vi "createNewArrayObject.vi"(8 "error in (no error)":errorcluster, 10 "arrayRef":refnum<vi>, 11 "Enum in":refnum<class "Enum.lvclass">) -> (0 "error out":errorcluster, 3 "Enum out":refnum<class "Enum.lvclass">)   [LabVIEW 2016, in "Enum.lvclass"]
uses:
  Enum.lvclass
  <vilib>/Utility/miscctls.llb/LVPointTypeDef.ctl
  Enum.lvclass/Enum.ctl
panel:
  in  "Enum":enum32{""}(ring)
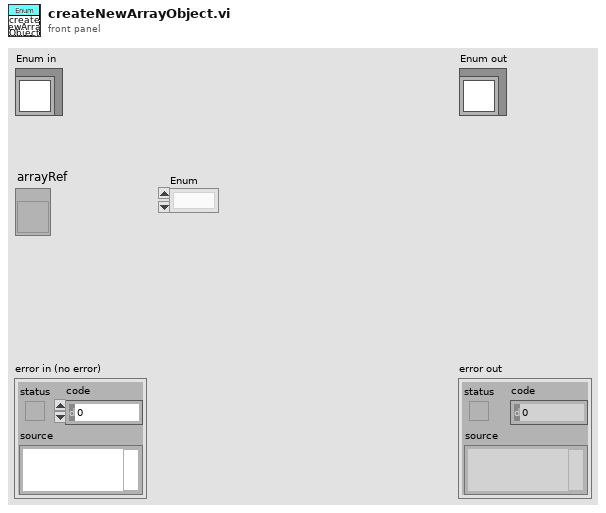
[diagram p1: front panel]
types:
  T1 = typedef "LVPointTypeDef.ctl" = cluster{"Horizontal":i16, "Vertical":i16}
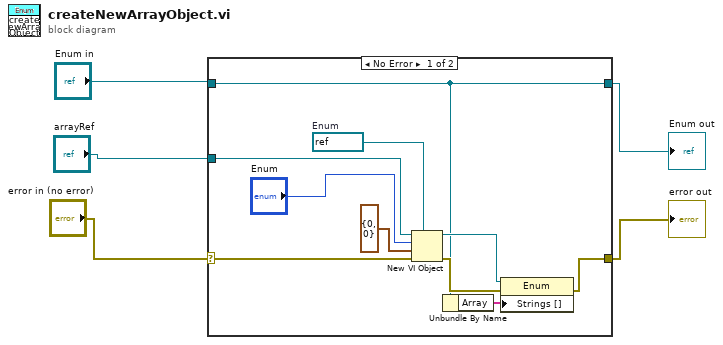
[diagram p0: block diagram]
diagram:
  n1 = case shown="No Error" "error in (no error)" {
    selector: "error in (no error)" -> [w11 w16]
    tunnel: "arrayRef" -> [w13 _]
    tunnel: [w12 w16] -> w3
    tunnel: [w8 w17] -> w4
    tunnel: "Enum in" -> [w8 w17]
    frame No Error {
      w9 = refnum<vi> refnum  # Enum
      n2 = New VI Object(vi object class=w9, owner refnum=w13, style="Enum", position/next to=T1 {"Horizontal"=0, "Vertical"=0} ("location"), 8:w11) -> (object refnum=w14:refnum<vi>, 0:w10:errorcluster)  [unwired: 3 in]
      n3 = Unbundle By Name(w8) -> ("Array"=w7:string[])
      n4 = property class="Enum"(reference=w14, error in=w10, "Strings []"=w7) -> (error out=w12:errorcluster)  [unwired: 1 out]
    }
    frame Error {
    }
  }
  "error out" <- w3
  "Enum out" <- w4
